vi "Create-load-file.vi"(8 "error in (no error)":errorcluster, 9 "Path type":bool, 10 "File path":path) -> (0 "error out":errorcluster, 3 "Load-file out":refnum<class "Load-file.lvclass">)   [LabVIEW 2013, in "Messages.lvlib" / "Load-file.lvclass"]
uses:
  Load-file.lvclass
  Base-messages.ctl
  Base-actions.ctl
  Action/Action.lvclass/Action.ctl
  Load-file.lvclass/Load-file.ctl
  Messages.lvlib
  Action/Action.lvclass
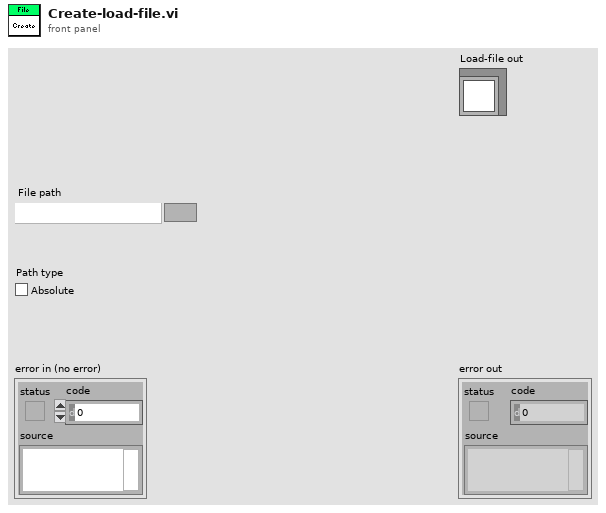
[diagram p1: front panel]
types:
  T1 = typedef "Messages.lvlib/Base-actions.ctl" = enum16{"Idle", "Initialize", "Load settings", "Load file", "Activate", "Start", "Pause", "Stop", "Repeat", "Reset", "Exit"}
  T2 = typedef "Messages.lvlib/Base-messages.ctl" = enum16{"Heartbeat", "Error", "Start client", "Stop client", "Get clients", "Query status", "Send status", "Action"}
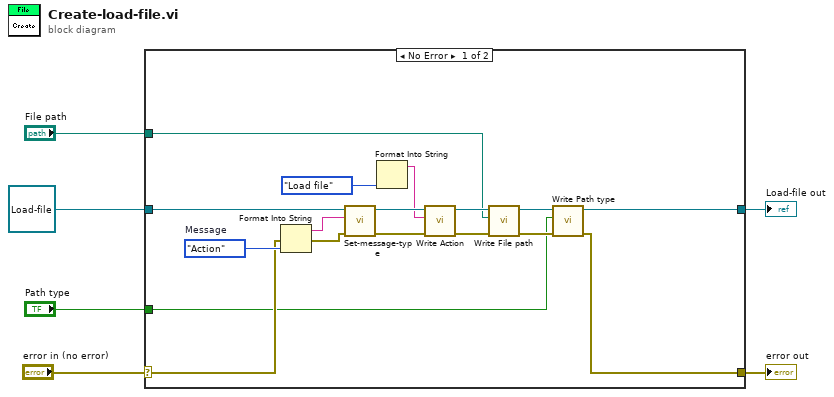
[diagram p0: block diagram]
diagram:
  n1 = case shown="No Error" "error in (no error)" {
    selector: "error in (no error)" -> [w19 w25]
    tunnel: [w12 w25] -> w5
    tunnel: [w9 w24] -> w4
    tunnel: refnum<class "Load-file.lvclass"> refnum ("Message in") -> [w23 w24]
    tunnel: "File path" -> [w8 _]
    tunnel: "Path type" -> [w7 _]
    frame No Error {
      w22 = Base-messages."Action"  # Message
      n2 = Format Into String(error in=w19, w22) -> (resulting string=w21:string, error out=w20:errorcluster)  [unwired: 2 in]
      n3 = call-dynamic "Set-message-type.vi"("error in (no error)"=w20, "Message type"=w21, "Message in"=w23) -> ("error out"=w17:errorcluster, "Message out"=w18:refnum<class "Load-file.lvclass">)  [unwired: 7 in]
      n4 = Format Into String(Base-actions."Load file" ("Action")) -> (resulting string=w15:string)  [unwired: 3 in, 1 out]
      n5 = call "Write Action.vi"("error in (no error)"=w17, "Action"=w15, "Action in"=w18) -> ("error out"=w14:errorcluster, "Action out"=w11:refnum<class "Load-file.lvclass">)  [unwired: 7 in]
      n6 = call "Write File path.vi"("error in (no error)"=w14, "File path"=w8, "Load-file in"=w11) -> ("error out"=w13:errorcluster, "Load-file out"=w10:refnum<class "Load-file.lvclass">)  [unwired: 7 in]
      n7 = call "Write Path type.vi"("error in (no error)"=w13, "Path type"=w7, "Load-file in"=w10) -> ("error out"=w12:errorcluster, "Load-file out"=w9:refnum<class "Load-file.lvclass">)  [unwired: 7 in]
    }
    frame Error {
    }
  }
  "error out" <- w5
  "Load-file out" <- w4
